vi "LXI Array to String.vi"(10 "LXI Triggers":bool[](array[boolean])=[TRUE, TRUE, TRUE, TRUE, TRUE, TRUE, TRUE, TRUE]) -> (2 "LXI Command String":string)   [LabVIEW 2012, in "Keysight B2980 Series.lvlib"]
doc: "Parse LXI Triggers array which contains 8 booleans to indicate the use of specified LXI Triggers to a comma separated string accepted by SCPI command."
uses:
  Keysight B2980 Series.lvlib
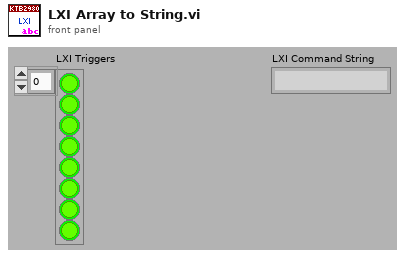
[diagram p1: front panel]
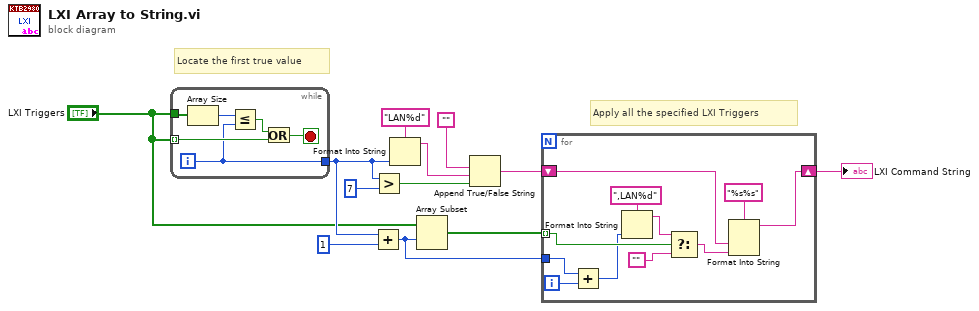
[diagram p0: block diagram]
diagram:
  # "Apply all the specified LXI Triggers"
  # "Locate the first true value"
  n1 = while {
    tunnel: "LXI Triggers" -> [w17] mode=indexing
    tunnel: [w14] -> w8
    tunnel: "LXI Triggers" -> [w18]
    i -> [w14]
    stop <- w16 stop-if-true
    n2 = Array Size(array=w18) -> (size(s)=w15:i32)
    n3 = Less Or Equal?(x=w15, y=w14) -> (x <= y?=w13:bool)
    n4 = Or(x=w13, y=w17) -> (x .or. y?=w16:bool)
  }
  n5 = Add(x=w8, y=1) -> (x+y=w9:i32)
  n6 = Greater?(x=w8, y=7) -> (0:w6:bool)
  n7 = Format Into String(format string="LAN%d", w8) -> (resulting string=w5:string)  [unwired: 2 in, 1 out]
  n8 = Array Subset(array="LXI Triggers", index=w9) -> (w11:bool[])  [unwired: 1 in]
  n9 = Append True/False String(1:w6, 2:w5, 3:"") -> (0:w4:string)  [unwired: 1 out]
  n10 = for {
    shift-right: [w22] -> w1
    shift-left: w4 -> [w20]
    tunnel: w11 -> [w26] mode=indexing
    tunnel: w9 -> [w23]
    i -> [w25]
    n11 = Add(x=w23, y=w25) -> (x+y=w24:i32)
    n12 = Format Into String(format string=",LAN%d", w24) -> (resulting string=w29:string)  [unwired: 2 in, 1 out]
    n13 = Select(t=w29, s=w26, f="") -> (s? t:f=w21:string)
    n14 = Format Into String(format string="%s%s", w20, w21) -> (resulting string=w22:string)  [unwired: 2 in, 1 out]
  }
  "LXI Command String" <- w1
